vi "Debug_Convert_Data_to_String.vi"(8 "error in (no error)":errorcluster, 11 "AB_Source_PackedItem in":refnum<class "AB_Source_PackedItem.lvclass">) -> (0 "error out":errorcluster, 1 "classData":string, 2 "sourceType":string, 3 "AB_Source_PackedItem out":refnum<class "AB_Source_PackedItem.lvclass">)   [LabVIEW 2020, in "AB_Source_PackedItem.lvclass"]
uses:
  <vilib>/AppBuilder/AB_Classes/Source/PackedItem/AB_Source_PackedItem.lvclass
  <vilib>/AppBuilder/AB_Classes/Source/AB_Source.lvclass
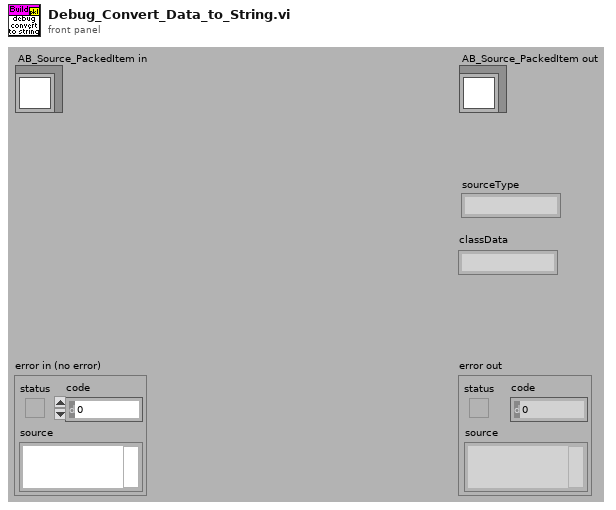
[diagram p1: front panel]
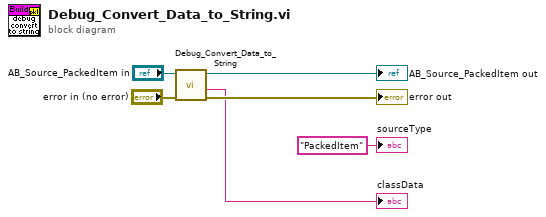
[diagram p0: block diagram]
diagram:
  n1 = call-parent "Debug_Convert_Data_to_String.vi"("error in (no error)"="error in (no error)", "AB_Source in"="AB_Source_PackedItem in") -> ("error out"=→"error out":errorcluster, "classData"=→"classData":string, "AB_Source out"=→"AB_Source_PackedItem out":refnum<class "AB_Source_PackedItem.lvclass">)  [unwired: 6 in, 1 out]
  "sourceType" <- "PackedItem" ("sourceType")
